vi "数字量Can请求发送.vi"(8 "第几组数据":u8, 10 "CANID":u32 format="%x", 11 "CANPort":u16) -> (2 "发送成功?":bool)   [LabVIEW 2010]
uses:
  全局量/全局_配置.vi
panel:
  in  "Data":u8[](array[numeric])
  in  "Send_MSG":T1(array[cluster])=[{"Flags"=4, "ID(HEX)"=0, "Data "=[0, 0, 0, 0, 0, 0, 0, 0]}, {"Flags"=4, "ID(HEX)"=0, "Data "=[0, 0, 0, 0, 0, 0, 0, 1]}, {"Flags"=4, "ID(HEX)"=0, "Data "=[0, 0, 0, 0, 0, 0, 0, 2]}, {"Flags"=4, "ID(HEX)"=0, "Data "=[0, 0, 0, 0, 0, 0, 0, 3]}, {"Flags"=4, "ID(HEX)"=0, "Data "=[0, 0, 0, 0, 0, 0, 0, 4]}, {"Flags"=4, "ID(HEX)"=0, "Data "=[0, 0, 0, 0, 0, 0, 0, 5]}, {"Flags"=4, "ID(HEX)"=0, "Data "=[0, 0, 0, 0, 0, 0, 0, 6]}, {"Flags"=4, "ID(HEX)"=0, "Data "=[0, 0, 0, 0, 0, 0, 0, 7]}, {"Flags"=4, "ID(HEX)"=0, "Data "=[0, 0, 0, 0, 0, 0, 0, 8]}, {"Flags"=4, "ID(HEX)"=0, "Data "=[0, 0, 0, 0, 0, 0, 0, 9]}, {"Flags"=4, "ID(HEX)"=0, "Data "=[0, 0, 0, 0, 0, 0, 1, 0]}, {"Flags"=4, "ID(HEX)"=0, "Data "=[0, 0, 0, 0, 0, 0, 1, 1]}, {"Flags"=4, "ID(HEX)"=0, "Data "=[0, 0, 0, 0, 0, 0, 1, 2]}, {"Flags"=4, "ID(HEX)"=0, "Data "=[0, 0, 0, 0, 0, 0, 1, 3]}, {"Flags"=4, "ID(HEX)"=0, "Data "=[0, 0, 0, 0, 0, 0, 1, 4]}, {"Flags"=4, "ID(HEX)"=0, "Data "=[0, 0, 0, 0, 0, 0, 1, 5]}, {"Flags"=4, "ID(HEX)"=0, "Data "=[0, 0, 0, 0, 0, 0, 1, 6]}, {"Flags"=4, "ID(HEX)"=0, "Data "=[0, 0, 0, 0, 0, 0, 1, 7]}, {"Flags"=4, "ID(HEX)"=0, "Data "=[0, 0, 0, 0, 0, 0, 1, 8]}, {"Flags"=4, "ID(HEX)"=0, "Data "=[0, 0, 0, 0, 0, 0, 1, 9]}, {"Flags"=4, "ID(HEX)"=0, "Data "=[0, 0, 0, 0, 0, 0, 2, 0]}, {"Flags"=4, "ID(HEX)"=0, "Data "=[0, 0, 0, 0, 0, 0, 2, 1]}, {"Flags"=4, "ID(HEX)"=0, "Data "=[0, 0, 0, 0, 0, 0, 2, 2]}, {"Flags"=4, "ID(HEX)"=0, "Data "=[0, 0, 0, 0, 0, 0, 2, 3]}, {"Flags"=4, "ID(HEX)"=0, "Data "=[0, 0, 0, 0, 0, 0, 2, 4]}, {"Flags"=4, "ID(HEX)"=0, "Data "=[0, 0, 0, 0, 0, 0, 2, 5]}, {"Flags"=4, "ID(HEX)"=0, "Data "=[0, 0, 0, 0, 0, 0, 2, 6]}, {"Flags"=4, "ID(HEX)"=0, "Data "=[0, 0, 0, 0, 0, 0, 2, 7]}, {"Flags"=4, "ID(HEX)"=0, "Data "=[0, 0, 0, 0, 0, 0, 2, 8]}, {"Flags"=4, "ID(HEX)"=0, "Data "=[0, 0, 0, 0, 0, 0, 2, 9]}, {"Flags"=4, "ID(HEX)"=0, "Data "=[0, 0, 0, 0, 0, 0, 3, 0]}, {"Flags"=4, "ID(HEX)"=0, "Data "=[0, 0, 0, 0, 0, 0, 3, 1]}, {"Flags"=4, "ID(HEX)"=0, "Data "=[0, 0, 0, 0, 0, 0, 3, 2]}, {"Flags"=4, "ID(HEX)"=0, "Data "=[0, 0, 0, 0, 0, 0, 3, 3]}, {"Flags"=4, "ID(HEX)"=0, "Data "=[0, 0, 0, 0, 0, 0, 3, 4]}, {"Flags"=4, "ID(HEX)"=0, "Data "=[0, 0, 0, 0, 0, 0, 3, 5]}, {"Flags"=4, "ID(HEX)"=0, "Data "=[0, 0, 0, 0, 0, 0, 3, 6]}, {"Flags"=4, "ID(HEX)"=0, "Data "=[0, 0, 0, 0, 0, 0, 3, 7]}, {"Flags"=4, "ID(HEX)"=0, "Data "=[0, 0, 0, 0, 0, 0, 3, 8]}, {"Flags"=4, "ID(HEX)"=0, "Data "=[0, 0, 0, 0, 0, 0, 3, 9]}, {"Flags"=4, "ID(HEX)"=0, "Data "=[0, 0, 0, 0, 0, 0, 4, 0]}, {"Flags"=4, "ID(HEX)"=0, "Data "=[0, 0, 0, 0, 0, 0, 4, 1]}, {"Flags"=4, "ID(HEX)"=0, "Data "=[0, 0, 0, 0, 0, 0, 4, 2]}, {"Flags"=4, "ID(HEX)"=0, "Data "=[0, 0, 0, 0, 0, 0, 4, 3]}, {"Flags"=4, "ID(HEX)"=0, "Data "=[0, 0, 0, 0, 0, 0, 4, 4]}, {"Flags"=4, "ID(HEX)"=0, "Data "=[0, 0, 0, 0, 0, 0, 4, 5]}, {"Flags"=4, "ID(HEX)"=0, "Data "=[0, 0, 0, 0, 0, 0, 4, 6]}, {"Flags"=4, "ID(HEX)"=0, "Data "=[0, 0, 0, 0, 0, 0, 4, 7]}, {"Flags"=4, "ID(HEX)"=0, "Data "=[0, 0, 0, 0, 0, 0, 4, 8]}, {"Flags"=4, "ID(HEX)"=0, "Data "=[0, 0, 0, 0, 0, 0, 4, 9]}, {"Flags"=4, "ID(HEX)"=0, "Data "=[0, 0, 0, 0, 0, 0, 5, 0]}, {"Flags"=4, "ID(HEX)"=0, "Data "=[0, 0, 0, 0, 0, 0, 5, 1]}, {"Flags"=4, "ID(HEX)"=0, "Data "=[0, 0, 0, 0, 0, 0, 5, 2]}, {"Flags"=4, "ID(HEX)"=0, "Data "=[0, 0, 0, 0, 0, 0, 5, 3]}, {"Flags"=4, "ID(HEX)"=0, "Data "=[0, 0, 0, 0, 0, 0, 5, 4]}, {"Flags"=4, "ID(HEX)"=0, "Data "=[0, 0, 0, 0, 0, 0, 5, 5]}, {"Flags"=4, "ID(HEX)"=0, "Data "=[0, 0, 0, 0, 0, 0, 5, 6]}, {"Flags"=4, "ID(HEX)"=0, "Data "=[0, 0, 0, 0, 0, 0, 5, 7]}, {"Flags"=4, "ID(HEX)"=0, "Data "=[0, 0, 0, 0, 0, 0, 5, 8]}, {"Flags"=4, "ID(HEX)"=0, "Data "=[0, 0, 0, 0, 0, 0, 5, 9]}, {"Flags"=4, "ID(HEX)"=0, "Data "=[0, 0, 0, 0, 0, 0, 6, 0]}, {"Flags"=4, "ID(HEX)"=0, "Data "=[0, 0, 0, 0, 0, 0, 6, 1]}, {"Flags"=4, "ID(HEX)"=0, "Data "=[0, 0, 0, 0, 0, 0, 6, 2]}, {"Flags"=4, "ID(HEX)"=0, "Data "=[0, 0, 0, 0, 0, 0, 6, 3]}, {"Flags"=4, "ID(HEX)"=0, "Data "=[0, 0, 0, 0, 0, 0, 6, 4]}, {"Flags"=4, "ID(HEX)"=0, "Data "=[0, 0, 0, 0, 0, 0, 6, 5]}, {"Flags"=4, "ID(HEX)"=0, "Data "=[0, 0, 0, 0, 0, 0, 6, 6]}, {"Flags"=4, "ID(HEX)"=0, "Data "=[0, 0, 0, 0, 0, 0, 6, 7]}, {"Flags"=4, "ID(HEX)"=0, "Data "=[0, 0, 0, 0, 0, 0, 6, 8]}, {"Flags"=4, "ID(HEX)"=0, "Data "=[0, 0, 0, 0, 0, 0, 6, 9]}, {"Flags"=4, "ID(HEX)"=0, "Data "=[0, 0, 0, 0, 0, 0, 7, 0]}, {"Flags"=4, "ID(HEX)"=0, "Data "=[0, 0, 0, 0, 0, 0, 7, 1]}, {"Flags"=4, "ID(HEX)"=0, "Data "=[0, 0, 0, 0, 0, 0, 7, 2]}, {"Flags"=4, "ID(HEX)"=0, "Data "=[0, 0, 0, 0, 0, 0, 7, 3]}, {"Flags"=4, "ID(HEX)"=0, "Data "=[0, 0, 0, 0, 0, 0, 7, 4]}, {"Flags"=4, "ID(HEX)"=0, "Data "=[0, 0, 0, 0, 0, 0, 7, 5]}, {"Flags"=4, "ID(HEX)"=0, "Data "=[0, 0, 0, 0, 0, 0, 7, 6]}, {"Flags"=4, "ID(HEX)"=0, "Data "=[0, 0, 0, 0, 0, 0, 7, 7]}, {"Flags"=4, "ID(HEX)"=0, "Data "=[0, 0, 0, 0, 0, 0, 7, 8]}, {"Flags"=4, "ID(HEX)"=0, "Data "=[0, 0, 0, 0, 0, 0, 7, 9]}, {"Flags"=4, "ID(HEX)"=0, "Data "=[0, 0, 0, 0, 0, 0, 8, 0]}, {"Flags"=4, "ID(HEX)"=0, "Data "=[0, 0, 0, 0, 0, 0, 8, 1]}, {"Flags"=4, "ID(HEX)"=0, "Data "=[0, 0, 0, 0, 0, 0, 8, 2]}, {"Flags"=4, "ID(HEX)"=0, "Data "=[0, 0, 0, 0, 0, 0, 8, 3]}, {"Flags"=4, "ID(HEX)"=0, "Data "=[0, 0, 0, 0, 0, 0, 8, 4]}, {"Flags"=4, "ID(HEX)"=0, "Data "=[0, 0, 0, 0, 0, 0, 8, 5]}, {"Flags"=4, "ID(HEX)"=0, "Data "=[0, 0, 0, 0, 0, 0, 8, 6]}, {"Flags"=4, "ID(HEX)"=0, "Data "=[0, 0, 0, 0, 0, 0, 8, 7]}, {"Flags"=4, "ID(HEX)"=0, "Data "=[0, 0, 0, 0, 0, 0, 8, 8]}, {"Flags"=4, "ID(HEX)"=0, "Data "=[0, 0, 0, 0, 0, 0, 8, 9]}, {"Flags"=4, "ID(HEX)"=0, "Data "=[0, 0, 0, 0, 0, 0, 9, 0]}, {"Flags"=4, "ID(HEX)"=0, "Data "=[0, 0, 0, 0, 0, 0, 9, 1]}, {"Flags"=4, "ID(HEX)"=0, "Data "=[0, 0, 0, 0, 0, 0, 9, 2]}, {"Flags"=4, "ID(HEX)"=0, "Data "=[0, 0, 0, 0, 0, 0, 9, 3]}, {"Flags"=4, "ID(HEX)"=0, "Data "=[0, 0, 0, 0, 0, 0, 9, 4]}, {"Flags"=4, "ID(HEX)"=0, "Data "=[0, 0, 0, 0, 0, 0, 9, 5]}, {"Flags"=4, "ID(HEX)"=0, "Data "=[0, 0, 0, 0, 0, 0, 9, 6]}, {"Flags"=4, "ID(HEX)"=0, "Data "=[0, 0, 0, 0, 0, 0, 9, 7]}, {"Flags"=4, "ID(HEX)"=0, "Data "=[0, 0, 0, 0, 0, 0, 9, 8]}, {"Flags"=4, "ID(HEX)"=0, "Data "=[0, 0, 0, 0, 0, 0, 9, 9]}] {"Data" format="%x"; "Flags" items=["MSG_STD"=0, "MSG_EXT"=4]; "ID(HEX)" format="%x"}
  out "Error out":errorcluster {"code" format="%.0x"}
  in  "WriteTimeOut":u32=5000 caption="ms"
  in  "Synchronization":i32(ring)=1 items=["Synchronization"=1, "Asynchronization"=0]
  # "同步异步"
  # "从1开始"
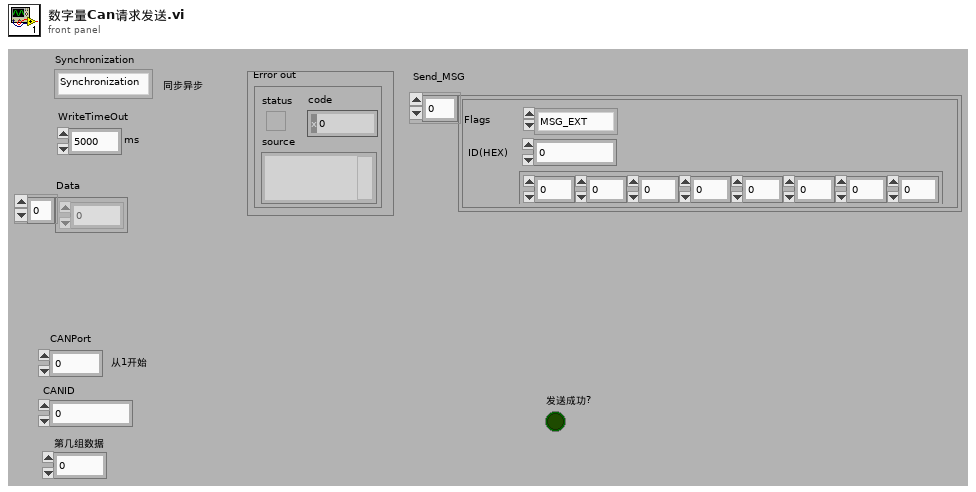
[diagram p1: front panel]
types:
  T1 = cluster{"Flags":u32, "ID(HEX)":u32, "Data ":u8[]}[]
  T2 = cluster{"Internal":u32, "InternalHigh":u32, "Offset":u32, "OffsetHigh":u32, "hEvent":u32}
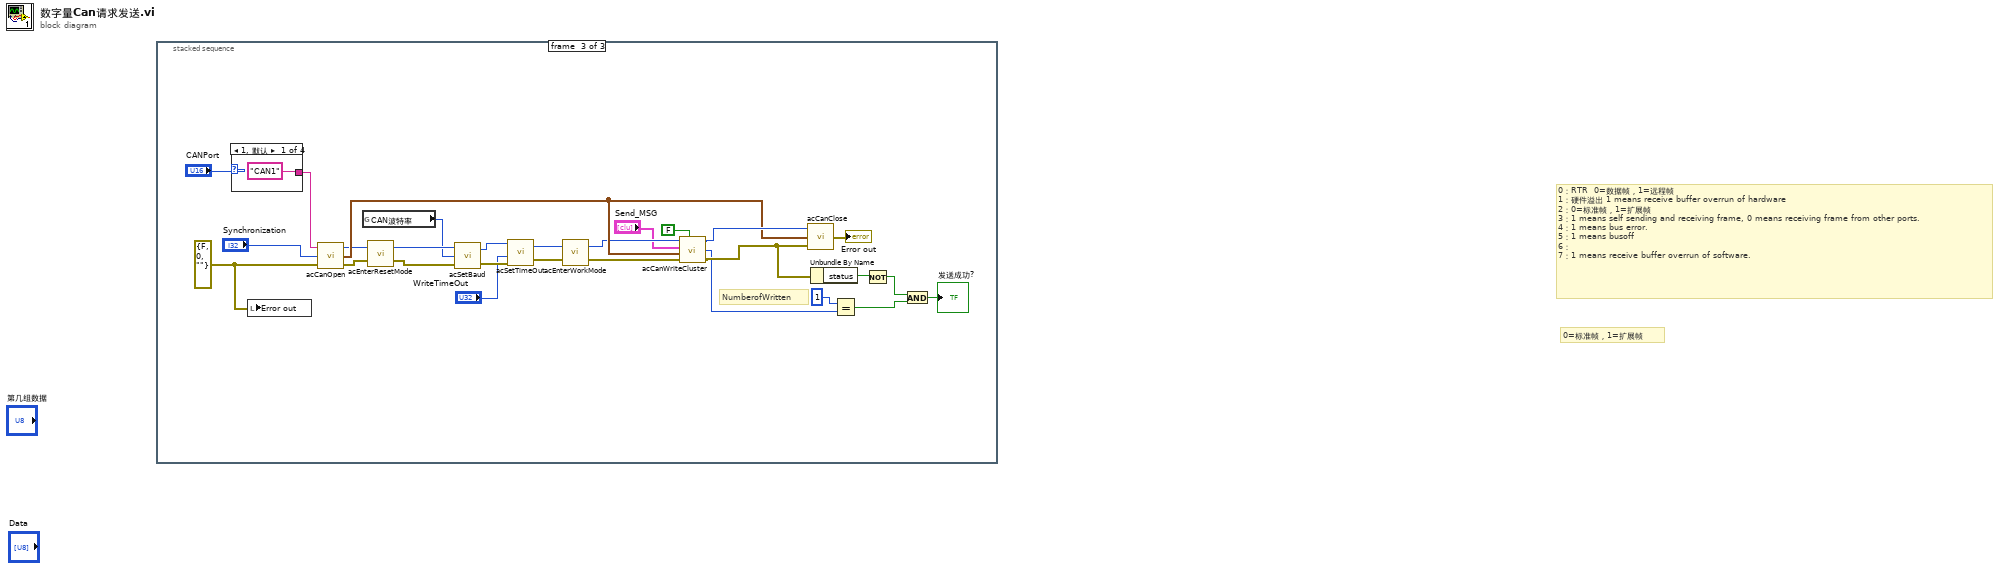
[diagram p0: block diagram]
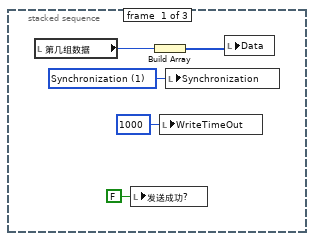
[diagram p2: hidden frame]
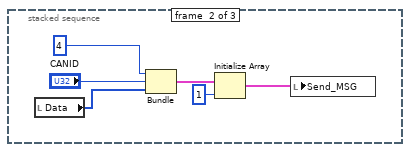
[diagram p3: hidden frame]
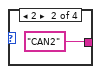
[diagram p4: hidden frame]
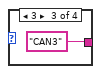
[diagram p5: hidden frame]
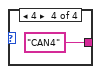
[diagram p6: hidden frame]
diagram:
  # "0=标准帧，1=扩展帧"
  # "0：RTR  0=数据帧，1=远程帧\n1：硬件溢出 1 means receive buffer overrun of hardware\n2：0=标准帧，1=扩展帧\n3：1 means self sending and receiving frame, 0 means receiving frame from other ports.\n4：1 means bus error.\n5：1 means busoff\n6：\n7：1 means receive buffer overrun of software."
  n1 = stacked-sequence {
    frame #0 {
      w3 = 1 items=["Synchronization"=1, "Asynchronization"=0] ("Synchronization")
      n2 = local read "第几组数据"() -> (w5:u8)
      n3 = local write "发送成功?"(FALSE ("发送成功?")) -> ()
      n4 = Build Array(w5) -> (w4:u8[])
      n5 = local write "WriteTimeOut"(u32 1000 ("WriteTimeOut")) -> ()
      n6 = local write "Synchronization"(w3) -> ()
      n7 = local write "Data"(w4) -> ()
    }
    frame #1 {
      n8 = local read "Data"() -> (w6:u8[])
      n9 = Bundle(u32 4, "CANID"="CANID", "Data"=w6) -> (w11:cluster{u32, "CANID":u32, "Data":u8[]})  [unwired: 1 in]
      n10 = Initialize Array(w11, 1 ("维数大小")) -> (w7:cluster{u32, "CANID":u32, "Data":u8[]}[])
      n11 = local write "Send_MSG"(w7) -> ()
    }
    frame #2 {
      w30 = errorcluster {"status"=FALSE, "code"=0, "source"=""} ("Error in")
      # "NumberofWritten"
      n12 = case shown="1, 默认" "CANPort" {
        tunnel: ["CAN1" "CAN2" "CAN3" "CAN4"] -> w22
        frame 1, Default {
        }
        frame 2 {
        }
        frame 3 {
        }
        frame 4 {
        }
      }
      n13 = local write "Error out"(w30) -> ()
      n14 = call "acCanOpen.vi"("Error in"=w30, "Synchronization"="Synchronization", "CANPort"=w22) -> ("Error out"=w27:errorcluster, "Overlapped"=w37:T2, "Handle"=w28:u32)
      n15 = global read "全局_配置.vi" "CAN波特率"() -> (w12:u16)
      n16 = call "acEnterResetMode.vi"("Error in"=w27, "Handle  in"=w28) -> ("Error out"=w35:errorcluster, "Handle out"=w34:u32)
      n17 = call "acSetBaud.vi"("Error in"=w35, "Baudrate"=w12, "Handle  in"=w34) -> ("Error out"=w36:errorcluster, "Handle out"=w24:u32)
      n18 = call "acSetTimeOut.vi"("Error in"=w36, "WriteTimeOut"="WriteTimeOut", "Handle  in"=w24) -> ("Error out"=w31:errorcluster, "Handle out"=w32:u32)  [unwired: 1 in]
      n19 = call "acEnterWorkMode.vi"("Error in"=w31, "Handle  in"=w32) -> ("Error out"=w26:errorcluster, "Handle out"=w25:u32)
      n20 = call "acCanWriteCluster.vi"("Handle  in"=w25, "MSG"="Send_MSG", "Overlapped"=w37, "Error in"=w26, "MSG_RTR"=FALSE) -> ("Handle out"=w38:u32, "NumberOfWritten"=w13:u32, "Error out"=w39:errorcluster)
      n21 = call "acCanClose.vi"("Error in"=w39, "Overlapped"=w37, "Handle  in"=w38) -> ("Error out"=→"Error out":errorcluster)
      n22 = Unbundle By Name(w39) -> ("status"=w18:bool)
      n23 = Equal?(x=u32 1, y=w13) -> (x = y?=w16:bool)
      n24 = Not(x=w18) -> (.not. x?=w19:bool)
      n25 = And(x=w19, y=w16) -> (x .and. y?=→"发送成功?":bool)
    }
  }
